vi "Load.vi"(8 "error in (no error)":errorcluster, 11 "Gantry in":refnum<class "Gantry Class.lvclass">) -> (0 "error out":errorcluster, 3 "PickupTool out":refnum<class "PickupTool Class.lvclass">)   [LabVIEW 2011, in "PickupTool Class.lvclass"]
uses:
  PickupTool Class.lvclass
  Gantry Class/Gantry Class.lvclass
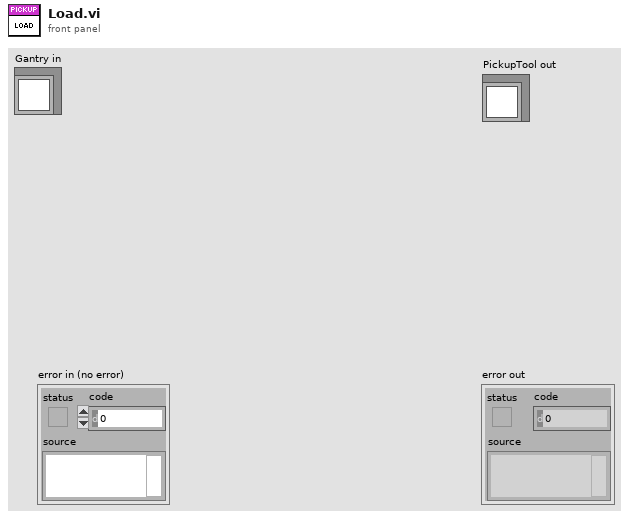
[diagram p1: front panel]
types:
  T1 = enum16{"None", "Grabber", "Picker", "Tool Setter"}
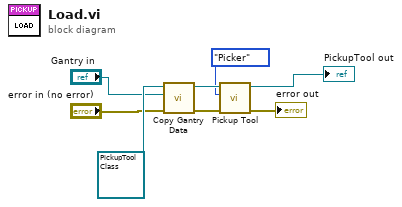
[diagram p0: block diagram]
diagram:
  n1 = call "Copy Gantry Data.vi"("error in (no error)"="error in (no error)", "Gantry Source"="Gantry in", "Gantry Dest"=refnum<class "PickupTool Class.lvclass"> refnum ("PickupTool Class in")) -> ("error out"=w7:errorcluster, "Gantry Result"=w8:refnum<class "PickupTool Class.lvclass">)  [unwired: 7 in]
  n2 = call-dynamic "Pickup Tool.vi"("error in (no error)"=w7, "Tool"=T1."Picker", "Gantry Class in"=w8) -> ("error out"=→"error out":errorcluster, "Gantry Class out"=→"PickupTool out":refnum<class "PickupTool Class.lvclass">)  [unwired: 7 in]
